vi "Update Sim.vi"(7 "Timings":T1, 8 "error in (no error)":errorcluster, 10 "Command":bool, 11 "ValveSimModule in":refnum<class "ValveSimModule.lvclass">) -> (0 "error out":errorcluster, 3 "ValveSimModule out":refnum<class "ValveSimModule.lvclass">)   [LabVIEW 2020, in "VolatusScratch.lvlib" / "ValveSimModule.lvclass"]
uses:
  ValveSimModule.lvclass
  ValveSimModule.lvclass/ValveSimModule.ctl
  Valve State.ctl
  Timings.ctl
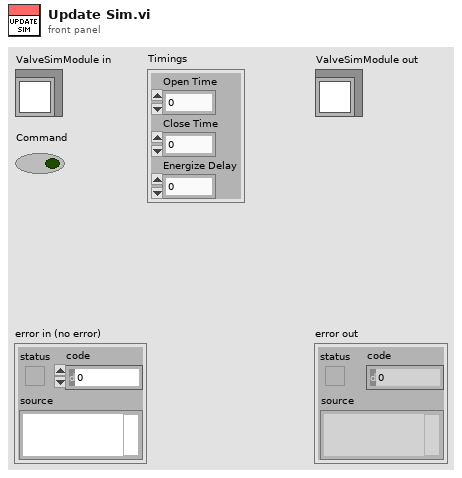
[diagram p1: front panel]
types:
  T1 = typedef "VolatusScratch.lvlib/ValveSimModule.lvclass/Timings.ctl" = cluster{"Open Time":dbl, "Close Time":dbl, "Energize Delay":dbl}
  T2 = typedef "VolatusScratch.lvlib/ValveSimModule.lvclass/Valve State.ctl" = enum16{"Closed", "Energize", "Open", "Opened", "Deenergize", "Close"}
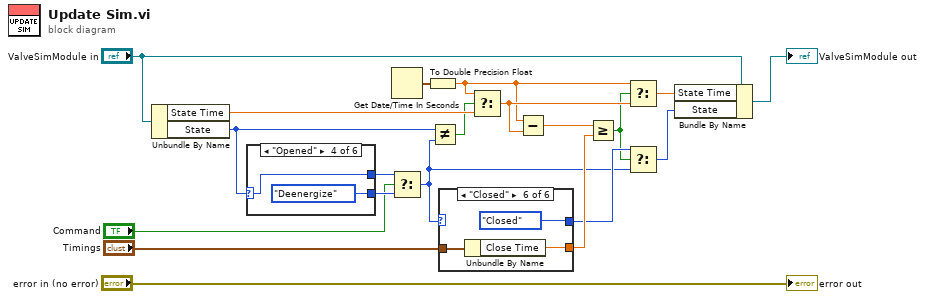
[diagram p0: block diagram]
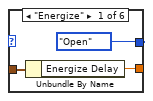
[diagram p2: hidden frame]
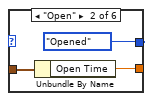
[diagram p3: hidden frame]
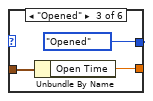
[diagram p4: hidden frame]
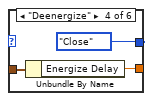
[diagram p5: hidden frame]
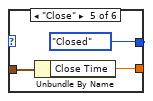
[diagram p6: hidden frame]
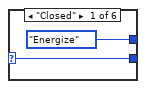
[diagram p7: hidden frame]
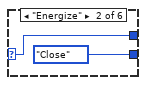
[diagram p8: hidden frame]
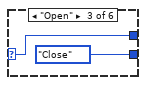
[diagram p9: hidden frame]
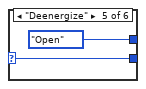
[diagram p10: hidden frame]
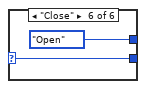
[diagram p11: hidden frame]
diagram:
  n1 = Unbundle By Name("ValveSimModule in") -> ("State Time"=w15:dbl, "State"=w14:T2)
  n2 = case shown="\"Opened\"" w14 {
    selector: w14 -> [w22 w24 w26 w28 w29 w31]
    tunnel: [w22 Valve_State."Close" ("State") Valve_State."Close" ("State") Valve_State."Deenergize" ("State") w29 w31] -> w17
    tunnel: [Valve_State."Energize" ("State") w24 w26 w28 Valve_State."Open" ("State") Valve_State."Open" ("State")] -> w18
    frame "Closed" {
    }
    frame "Energize" {
    }
    frame "Open" {
    }
    frame "Opened" {
    }
    frame "Deenergize" {
    }
    frame "Close" {
    }
  }
  n3 = Get Date/Time In Seconds() -> (seconds since 1Jan1904=w19:timestamp)
  n4 = Select(t=w18, s="Command", f=w17) -> (s? t:f=w8:T2)
  n5 = To Double Precision Float(number=w19) -> (double precision float=w6:dbl)
  n6 = Not Equal?(x=w14, y=w8) -> (x != y?=w13:bool)
  n7 = case shown="\"Closed\"" w8 {
    tunnel: "Timings" -> [w35 w38 w41 w44 w47 w50]
    tunnel: [w34 w37 w40 w43 w46 w49] -> w10
    tunnel: [Valve_State."Open" ("State") Valve_State."Opened" ("State") Valve_State."Opened" ("State") Valve_State."Close" ("State") Valve_State."Closed" ("State") Valve_State."Closed" ("State")] -> w9
    frame "Energize" {
      n8 = Unbundle By Name(w35) -> ("Energize Delay"=w34:dbl)
    }
    frame "Open" {
      n9 = Unbundle By Name(w38) -> ("Open Time"=w37:dbl)
    }
    frame "Opened" {
      n10 = Unbundle By Name(w41) -> ("Open Time"=w40:dbl)
    }
    frame "Deenergize" {
      n11 = Unbundle By Name(w44) -> ("Energize Delay"=w43:dbl)
    }
    frame "Close" {
      n12 = Unbundle By Name(w47) -> ("Close Time"=w46:dbl)
    }
    frame "Closed" {
      n13 = Unbundle By Name(w50) -> ("Close Time"=w49:dbl)
    }
  }
  n14 = Select(t=w6, s=w13, f=w15) -> (s? t:f=w7:dbl)
  n15 = Subtract(x=w6, y=w7) -> (x-y=w11:dbl)
  n16 = Greater Or Equal?(x=w11, y=w10) -> (x >= y?=w5:bool)
  n17 = Select(t=w6, s=w5, f=w7) -> (s? t:f=w4:dbl)
  n18 = Select(t=w9, s=w5, f=w8) -> (s? t:f=w3:T2)
  n19 = Bundle By Name(cluster="ValveSimModule in", "State Time"=w4, "State"=w3) -> (→"ValveSimModule out":refnum<class "ValveSimModule.lvclass">)
  "error out" <- "error in (no error)"
